vi "Autonomous Independent.vi"   [LabVIEW 2017] (continued)
                  n1739 = call "PID Distance.vi"("Distance"=225.0, "Angle"=0.0, "RightEncoder"=w5983, "LeftEncoder"=w5984, "GyroDevRef"=w5985, "RobotDriveDevRef"=w5986) -> ("RightEncoder 2"=w5987:T11, "LeftEncoder 2"=w5988:T11, "GyroDevRef 2"=w5989:T8, "RobotDriveDevRef 2"=w5990:T1)  [unwired: 2 in]
                }
                frame #1 {
                  n1740 = call "PID turning.vi"("Angle"=-90.0, "GyroDevRef"=w6002, "RobotDriveDevRef"=w6001) -> ("GyroDevRef 2"=w5999:T8, "RobotDriveDevRef 2"=w6000:T1)  [unwired: 7 in]
                }
                frame #2 {
                  n1741 = call <vilib>:"WPI_EncoderReset.vi"("EncoderDevRef"=w6011) -> ("EncoderDevRef"=w6009:T11)  [unwired: 9 in, 1 out]
                  n1742 = Wait (ms)(milliseconds to wait=u32 10) -> ()  [unwired: 1 out]
                  n1743 = call <vilib>:"WPI_EncoderReset.vi"("EncoderDevRef"=w6012) -> ("EncoderDevRef"=w6010:T11)  [unwired: 9 in, 1 out]
                }
                frame #3 {
                  n1744 = global read "Robot Global Data.vi" "Axes"() -> (w6024:dbl[])
                  n1745 = call "PID Distance.vi"("Distance"=199.0, "Angle"=-90.0, "RightEncoder"=w6017, "LeftEncoder"=w6018, "GyroDevRef"=w6019, "RobotDriveDevRef"=w6020) -> ("RightEncoder 2"=w6014:T11, "LeftEncoder 2"=w6013:T11, "GyroDevRef 2"=w6016:T8, "RobotDriveDevRef 2"=w6015:T1)  [unwired: 2 in]
                  n1746 = global write "Robot Global Data.vi" "Lift_Position"(2.0) -> ()
                  n1747 = Array To Cluster(array=w6024) -> (cluster=w6023:T15)
                  n1748 = Bundle By Name(cluster=w6023, "Axes[1]"=-1.0) -> (w6022:T15)
                  n1749 = Cluster To Array(cluster=w6022) -> (array=w6021:dbl[])
                  n1750 = global write "Robot Global Data.vi" "Axes"(w6021) -> ()
                }
                frame #4 {
                  n1751 = call "PID turning.vi"("Angle"=0.0, "GyroDevRef"=w6031, "RobotDriveDevRef"=w6032) -> ("GyroDevRef 2"=w6029:T8, "RobotDriveDevRef 2"=w6030:T1)  [unwired: 7 in]
                }
                frame #5 {
                  n1752 = call <vilib>:"WPI_EncoderReset.vi"("EncoderDevRef"=w6037) -> ("EncoderDevRef"=w6040:T11)  [unwired: 9 in, 1 out]
                  n1753 = call <vilib>:"WPI_EncoderReset.vi"("EncoderDevRef"=w6036) -> ("EncoderDevRef"=w6039:T11)  [unwired: 9 in, 1 out]
                }
                frame #6 {
                  n1754 = call "PID Distance.vi"("Distance"=40.0, "Angle"=0.0, "RightEncoder"=w6047, "LeftEncoder"=w6048, "GyroDevRef"=w6050, "RobotDriveDevRef"=w6049) -> ("RightEncoder 2"=w6043:T11, "LeftEncoder 2"=w6044:T11, "GyroDevRef 2"=w6045:T8, "RobotDriveDevRef 2"=w6046:T1)  [unwired: 2 in]
                  n1755 = global write "Robot Global Data.vi" "Lift_Position"(3.0) -> ()
                }
                frame #7 {
                  n1756 = call "PID turning.vi"("Angle"=20.0, "GyroDevRef"=w6054, "RobotDriveDevRef"=w6057) -> ("GyroDevRef 2"=w6053:T8, "RobotDriveDevRef 2"=w6056:T1)  [unwired: 7 in]
                }
                frame #8 {
                  n1757 = call <vilib>:"WPI_EncoderReset.vi"("EncoderDevRef"=w6063) -> ("EncoderDevRef"=w6061:T11)  [unwired: 9 in, 1 out]
                  n1758 = call <vilib>:"WPI_EncoderReset.vi"("EncoderDevRef"=w6062) -> ("EncoderDevRef"=w6060:T11)  [unwired: 9 in, 1 out]
                }
                frame #9 {
                  w6077 = 0.0 ("Left axis value")
                  n1759 = global read "Robot Global Data.vi" "Axes"() -> (w6072:dbl[])
                  n1760 = Wait (ms)(milliseconds to wait=u32 300) -> ()  [unwired: 1 out]
                  n1761 = Array To Cluster(array=w6072) -> (cluster=w6071:T15)
                  n1762 = Bundle By Name(cluster=w6071, "Axes[1]"=0.25) -> (w6074:T15)
                  n1763 = Cluster To Array(cluster=w6074) -> (array=w6073:dbl[])
                  n1764 = call <vilib>:"WPI_RobotDriveTankDrive.vi"("Right axis value"=w6077, "Left axis value"=w6077, "RobotDriveDevRef"=w6076) -> ("RobotDriveDevRef"=w6070:T1)  [unwired: 6 in, 2 out]
                  n1765 = global write "Robot Global Data.vi" "Axes"(w6073) -> ()
                }
                frame #10 {
                  n1766 = global write "Robot Global Data.vi" "Current State"(FALSE ("Current State")) -> ()
                  n1767 = Wait (ms)(milliseconds to wait=u32 400) -> ()  [unwired: 1 out]
                }
                frame #11 {
                  n1768 = global read "Robot Global Data.vi" "Axes"() -> (w6094:dbl[])
                  n1769 = call "PID Distance.vi"("Distance"=-20.0, "Angle"=20.0, "RightEncoder"=w6095, "LeftEncoder"=w6096, "GyroDevRef"=w6084, "RobotDriveDevRef"=w6085) -> ("RightEncoder 2"=w6086:T11, "LeftEncoder 2"=w6087:T11, "GyroDevRef 2"=w6088:T8, "RobotDriveDevRef 2"=w6089:T1)  [unwired: 2 in]
                  n1770 = Array To Cluster(array=w6094) -> (cluster=w6093:T15)
                  n1771 = Bundle By Name(cluster=w6093, "Axes[1]"=-1.0) -> (w6092:T15)
                  n1772 = Cluster To Array(cluster=w6092) -> (array=w6091:dbl[])
                  n1773 = global write "Robot Global Data.vi" "Axes"(w6091) -> ()
                }
                frame #12 {
                  n1774 = global write "Robot Global Data.vi" "Lift_Position"(1.0) -> ()
                }
                frame #13 {
                  n1775 = case shown="\"L\"" w6104 {
                    tunnel: w6108 -> [w6120 w6196 _]
                    tunnel: w6107 -> [w6119 w6195 _]
                    tunnel: w6106 -> [w6118 w6193 _]
                    tunnel: w6105 -> [w6117 w6194 _]
                    frame "R" {
                      n1776 = flat-sequence {
                        tunnel: w6120 -> [w6129]
                        tunnel: w6119 -> [w6128]
                        tunnel: [w6131] -> w6126
                        tunnel: [w6130] -> w6125
                        tunnel: w6126 -> [w6138]
                        tunnel: w6125 -> [w6137]
                        tunnel: [w6138] -> w6121
                        tunnel: [w6137] -> w6122
                        tunnel: [w6135] -> w6123
                        tunnel: [w6134] -> w6124
                        tunnel: w6118 -> [w6133]
                        tunnel: w6117 -> [w6132]
                        tunnel: w6124 -> [w6139]
                        tunnel: w6123 -> [w6140]
                        tunnel: w6122 -> [w6143]
                        tunnel: w6121 -> [w6144]
                        tunnel: [w6142] -> w6116
                        tunnel: [w6141] -> w6114
                        tunnel: [w6140] -> w6112
                        tunnel: [w6139] -> w6110
                        tunnel: w6116 -> [w6172]
                        tunnel: [w6172] -> w6115
                        tunnel: w6114 -> [w6171]
                        tunnel: [w6171] -> w6113
                        tunnel: w6112 -> [w6170]
                        tunnel: [w6168] -> w6111
                        tunnel: w6110 -> [w6169]
                        tunnel: [w6167] -> w6109
                        tunnel: w6115 -> [w6176]
                        tunnel: w6113 -> [w6175]
                        tunnel: w6111 -> [w6174]
                        tunnel: w6109 -> [w6173]
                        frame #0 {
                          n1777 = call "PID turning.vi"("Angle"=170.0, "GyroDevRef"=w6128, "RobotDriveDevRef"=w6129) -> ("GyroDevRef 2"=w6130:T8, "RobotDriveDevRef 2"=w6131:T1)  [unwired: 7 in]
                        }
                        frame #1 {
                          n1778 = call <vilib>:"WPI_EncoderReset.vi"("EncoderDevRef"=w6133) -> ("EncoderDevRef"=w6134:T11)  [unwired: 9 in, 1 out]
                          n1779 = Wait (ms)(milliseconds to wait=u32 10) -> ()  [unwired: 1 out]
                          n1780 = call <vilib>:"WPI_EncoderReset.vi"("EncoderDevRef"=w6132) -> ("EncoderDevRef"=w6135:T11)  [unwired: 9 in, 1 out]
                        }
                        frame #2 {
                          n1781 = global read "Robot Global Data.vi" "Axes"() -> (w6151:dbl[])
                          n1782 = Wait (ms)(milliseconds to wait=u32 400) -> ()  [unwired: 1 out]
                          n1783 = Array To Cluster(array=w6151) -> (cluster=w6152:T15)
                          n1784 = global read "Robot Global Data.vi" "PIXY Output"() -> (w6145:T16)
                          n1785 = Bundle By Name(cluster=w6152, "Axes[1]"=1.0) -> (w6153:T15)
                          n1786 = Unbundle By Name(w6145) -> ("SIGNATURE NUMBER"=w6148:u16)
                          n1787 = global read "Robot Global Data.vi" "Cube Signature"() -> (w6147:dbl)
                          n1788 = Equal?(x=w6148, y=w6147) -> (x = y?=w6146:bool)
                          n1789 = Cluster To Array(cluster=w6153) -> (array=w6154:dbl[])
                          n1790 = global write "Robot Global Data.vi" "Axes"(w6154) -> ()
                          n1791 = case shown="False" w6146 {
                            tunnel: [w6161 w6164] -> w6141
                            tunnel: [w6162 w6163] -> w6142
                            tunnel: w6144 -> [w6156 w6163]
                            tunnel: w6143 -> [w6155 w6164]
                            frame True {
                              n1792 = call <vilib>:"WPI_GyroGetAngle.vi"("GyroDevRef"=w6155) -> ("Angle"=w6160:dbl, "GyroDevRef"=w6161:T8)  [unwired: 6 in, 3 out]
                              n1793 = In Range and Coerce(upper limit=170.0, x=w6160, lower limit=110.0) -> (coerced(x)=w6159:dbl)  [unwired: 1 out]
                              n1794 = global write "Robot Global Data.vi" "Tracked Angle"(w6159) -> ()
                              n1795 = call "PID vision.vi"("RobotDriveDevRef in"=w6156) -> ("RobotDriveDevRef out"=w6162:T1)  [unwired: 9 in, 1 out]
                            }
                            frame False {
                              n1796 = global write "Robot Global Data.vi" "Tracked Angle"(170.0) -> ()
                            }
                          }
                        }
                        frame #3 {
                          n1797 = call <vilib>:"WPI_EncoderReset.vi"("EncoderDevRef"=w6169) -> ("EncoderDevRef"=w6167:T11)  [unwired: 9 in, 1 out]
                          n1798 = Wait (ms)(milliseconds to wait=u32 10) -> ()  [unwired: 1 out]
                          n1799 = call <vilib>:"WPI_EncoderReset.vi"("EncoderDevRef"=w6170) -> ("EncoderDevRef"=w6168:T11)  [unwired: 9 in, 1 out]
                        }
                        frame #4 {
                          n1800 = global read "Robot Global Data.vi" "Tracked Angle"() -> (w6177:dbl)
                          n1801 = call "PID Distance.vi"("Distance"=50.0, "Angle"=w6177, "RightEncoder"=w6173, "LeftEncoder"=w6174, "GyroDevRef"=w6175, "RobotDriveDevRef"=w6176) -> ()  [unwired: 2 in, 4 out]
                        }
                        frame #5 {
                          n1802 = global write "Robot Global Data.vi" "Current State"(TRUE ("Current State")) -> ()
                          n1803 = Wait (ms)(milliseconds to wait=u32 300) -> ()  [unwired: 1 out]
                        }
                      }
                    }
                    frame "L" {
                      n1804 = flat-sequence {
                        tunnel: w6196 -> [w6213]
                        tunnel: w6195 -> [w6212]
                        tunnel: [w6215] -> w6210
                        tunnel: [w6214] -> w6209
                        tunnel: w6210 -> [w6222]
                        tunnel: w6209 -> [w6221]
                        tunnel: [w6222] -> w6205
                        tunnel: [w6221] -> w6206
                        tunnel: [w6219] -> w6207
                        tunnel: [w6218] -> w6208
                        tunnel: w6193 -> [w6217]
                        tunnel: w6194 -> [w6216]
                        tunnel: w6208 -> [w6223]
                        tunnel: w6207 -> [w6224]
                        tunnel: w6206 -> [w6227]
                        tunnel: w6205 -> [w6228]
                        tunnel: [w6226] -> w6204
                        tunnel: [w6225] -> w6203
                        tunnel: [w6224] -> w6202
                        tunnel: [w6223] -> w6201
                        tunnel: w6204 -> [w6256]
                        tunnel: [w6256] -> w6200
                        tunnel: w6203 -> [w6255]
                        tunnel: [w6255] -> w6199
                        tunnel: w6202 -> [w6254]
                        tunnel: [w6252] -> w6198
                        tunnel: w6201 -> [w6253]
                        tunnel: [w6251] -> w6197
                        tunnel: w6200 -> [w6264]
                        tunnel: w6199 -> [w6263]
                        tunnel: w6198 -> [w6262]
                        tunnel: w6197 -> [w6261]
                        tunnel: [w6260] -> w6190
                        tunnel: [w6259] -> w6187
                        tunnel: [w6258] -> w6184
                        tunnel: [w6257] -> w6181
                        tunnel: [w6270] -> w6191
                        tunnel: w6190 -> [w6270]
                        tunnel: [w6269] -> w6188
                        tunnel: w6187 -> [w6269]
                        tunnel: [w6268] -> w6185
                        tunnel: w6184 -> [w6268]
                        tunnel: [w6267] -> w6182
                        tunnel: w6181 -> [w6267]
                        tunnel: [w6276] -> w6192
                        tunnel: w6191 -> [w6276]
                        tunnel: [w6275] -> w6189
                        tunnel: w6188 -> [w6275]
                        tunnel: [w6274] -> w6186
                        tunnel: w6185 -> [w6274]
                        tunnel: [w6273] -> w6183
                        tunnel: w6182 -> [w6273]
                        tunnel: w6192 -> [w6287]
                        tunnel: w6189 -> [w6286]
                        tunnel: w6186 -> [w6285]
                        tunnel: w6183 -> [w6284]
                        frame #0 {
                          n1805 = call "PID turning.vi"("Angle"=170.0, "GyroDevRef"=w6212, "RobotDriveDevRef"=w6213) -> ("GyroDevRef 2"=w6214:T8, "RobotDriveDevRef 2"=w6215:T1)  [unwired: 7 in]
                        }
                        frame #1 {
                          n1806 = call <vilib>:"WPI_EncoderReset.vi"("EncoderDevRef"=w6217) -> ("EncoderDevRef"=w6218:T11)  [unwired: 9 in, 1 out]
                          n1807 = Wait (ms)(milliseconds to wait=u32 10) -> ()  [unwired: 1 out]
                          n1808 = call <vilib>:"WPI_EncoderReset.vi"("EncoderDevRef"=w6216) -> ("EncoderDevRef"=w6219:T11)  [unwired: 9 in, 1 out]
                        }
                        frame #2 {
                          n1809 = global read "Robot Global Data.vi" "Axes"() -> (w6235:dbl[])
                          n1810 = Wait (ms)(milliseconds to wait=u32 400) -> ()  [unwired: 1 out]
                          n1811 = Array To Cluster(array=w6235) -> (cluster=w6236:T15)
                          n1812 = global read "Robot Global Data.vi" "PIXY Output"() -> (w6229:T16)
                          n1813 = Bundle By Name(cluster=w6236, "Axes[1]"=1.0) -> (w6237:T15)
                          n1814 = Unbundle By Name(w6229) -> ("SIGNATURE NUMBER"=w6232:u16)
                          n1815 = global read "Robot Global Data.vi" "Cube Signature"() -> (w6231:dbl)
                          n1816 = Equal?(x=w6232, y=w6231) -> (x = y?=w6230:bool)
                          n1817 = Cluster To Array(cluster=w6237) -> (array=w6238:dbl[])
                          n1818 = global write "Robot Global Data.vi" "Axes"(w6238) -> ()
                          n1819 = case shown="True" w6230 {
                            tunnel: [w6245 w6248] -> w6225
                            tunnel: [w6246 w6247] -> w6226
                            tunnel: w6228 -> [w6240 w6247]
                            tunnel: w6227 -> [w6239 w6248]
                            frame True {
                              n1820 = call <vilib>:"WPI_GyroGetAngle.vi"("GyroDevRef"=w6239) -> ("Angle"=w6244:dbl, "GyroDevRef"=w6245:T8)  [unwired: 6 in, 3 out]
                              n1821 = In Range and Coerce(upper limit=170.0, x=w6244, lower limit=155.0) -> (coerced(x)=w6243:dbl)  [unwired: 1 out]
                              n1822 = global write "Robot Global Data.vi" "Tracked Angle"(w6243) -> ()
                              n1823 = call "PID vision.vi"("RobotDriveDevRef in"=w6240) -> ("RobotDriveDevRef out"=w6246:T1)  [unwired: 9 in, 1 out]
                            }
                            frame False {
                              n1824 = global write "Robot Global Data.vi" "Tracked Angle"(170.0) -> ()
                            }
                          }
                        }
                        frame #3 {
                          n1825 = call <vilib>:"WPI_EncoderReset.vi"("EncoderDevRef"=w6253) -> ("EncoderDevRef"=w6251:T11)  [unwired: 9 in, 1 out]
                          n1826 = Wait (ms)(milliseconds to wait=u32 10) -> ()  [unwired: 1 out]
                          n1827 = call <vilib>:"WPI_EncoderReset.vi"("EncoderDevRef"=w6254) -> ("EncoderDevRef"=w6252:T11)  [unwired: 9 in, 1 out]
                        }
                        frame #4 {
                          n1828 = global read "Robot Global Data.vi" "Tracked Angle"() -> (w6265:dbl)
                          n1829 = call "PID Distance.vi"("Distance"=50.0, "Angle"=w6265, "RightEncoder"=w6261, "LeftEncoder"=w6262, "GyroDevRef"=w6263, "RobotDriveDevRef"=w6264) -> ("RightEncoder 2"=w6257:T11, "LeftEncoder 2"=w6258:T11, "GyroDevRef 2"=w6259:T8, "RobotDriveDevRef 2"=w6260:T1)  [unwired: 2 in]
                        }
                        frame #5 {
                          n1830 = global write "Robot Global Data.vi" "Current State"(TRUE ("Current State")) -> ()
                          n1831 = Wait (ms)(milliseconds to wait=u32 500) -> ()  [unwired: 1 out]
                        }
                        frame #6 {
                          n1832 = global read "Robot Global Data.vi" "Axes"() -> (w6282:dbl[])
                          n1833 = global write "Robot Global Data.vi" "Lift_Position"(2.0) -> ()
                          n1834 = Wait (ms)(milliseconds to wait=u32 400) -> ()  [unwired: 1 out]
                          n1835 = Array To Cluster(array=w6282) -> (cluster=w6281:T15)
                          n1836 = Bundle By Name(cluster=w6281, "Axes[1]"=-1.0) -> (w6280:T15)
                          n1837 = Cluster To Array(cluster=w6280) -> (array=w6279:dbl[])
                          n1838 = global write "Robot Global Data.vi" "Axes"(w6279) -> ()
                        }
                        frame #7 {
                          n1839 = global read "Robot Global Data.vi" "Tracked Angle"() -> (w6288:dbl)
                          n1840 = call "PID Distance.vi"("Distance"=66.0, "Angle"=w6288, "RightEncoder"=w6284, "LeftEncoder"=w6285, "GyroDevRef"=w6286, "RobotDriveDevRef"=w6287) -> ()  [unwired: 2 in, 4 out]
                        }
                        frame #8 {
                          n1841 = global read "Robot Global Data.vi" "Axes"() -> (w6295:dbl[])
                          n1842 = Wait (ms)(milliseconds to wait=u32 200) -> ()  [unwired: 1 out]
                          n1843 = Array To Cluster(array=w6295) -> (cluster=w6294:T15)
                          n1844 = Bundle By Name(cluster=w6294, "Axes[1]"=0.5) -> (w6293:T15)
                          n1845 = Cluster To Array(cluster=w6293) -> (array=w6292:dbl[])
                          n1846 = global write "Robot Global Data.vi" "Axes"(w6292) -> ()
                        }
                        frame #9 {
                          n1847 = global write "Robot Global Data.vi" "Current State"(FALSE ("Current State")) -> ()
                        }
                      }
                    }
                    frame Default {
                    }
                  }
                }
              }
            }
            frame "R" {
              n1848 = flat-sequence {
                tunnel: [w6362] -> w6350
                tunnel: [w6361] -> w6351
                tunnel: [w6359] -> w6352
                tunnel: [w6360] -> w6353
                tunnel: w6309 -> [w6358]
                tunnel: w6308 -> [w6357]
                tunnel: w6307 -> [w6356]
                tunnel: w6306 -> [w6355]
                tunnel: [w6382] -> w6349
                tunnel: w6353 -> [w6378]
                tunnel: w6352 -> [w6379]
                tunnel: w6351 -> [w6381]
                tunnel: w6350 -> [w6383]
                tunnel: [w6380] -> w6348
                tunnel: [w6379] -> w6347
                tunnel: [w6378] -> w6346
                tunnel: w6349 -> [w6393]
                tunnel: [w6393] -> w6345
                tunnel: w6348 -> [w6392]
                tunnel: [w6392] -> w6344
                tunnel: [w6391] -> w6343
                tunnel: [w6390] -> w6342
                tunnel: w6347 -> [w6388]
                tunnel: w6346 -> [w6387]
                tunnel: w6345 -> [w6399]
                tunnel: [w6397] -> w6341
                tunnel: w6344 -> [w6398]
                tunnel: [w6396] -> w6340
                tunnel: w6343 -> [w6401]
                tunnel: w6342 -> [w6400]
                tunnel: [w6395] -> w6339
                tunnel: [w6394] -> w6338
                tunnel: w6341 -> [w6408]
                tunnel: [w6407] -> w6337
                tunnel: [w6406] -> w6336
                tunnel: w6340 -> [w6406]
                tunnel: [w6405] -> w6335
                tunnel: w6339 -> [w6405]
                tunnel: [w6404] -> w6334
                tunnel: w6338 -> [w6404]
                tunnel: [w6419] -> w6333
                tunnel: w6337 -> [w6419]
                tunnel: [w6418] -> w6332
                tunnel: w6336 -> [w6418]
                tunnel: [w6417] -> w6331
                tunnel: w6335 -> [w6417]
                tunnel: [w6416] -> w6330
                tunnel: w6334 -> [w6416]
                tunnel: w6333 -> [w6424]
                tunnel: w6332 -> [w6425]
                tunnel: [w6425] -> w6329
                tunnel: [w6424] -> w6328
                tunnel: [w6423] -> w6327
                tunnel: w6331 -> [w6423]
                tunnel: [w6422] -> w6326
                tunnel: w6330 -> [w6422]
                tunnel: [w6438] -> w6325
                tunnel: w6329 -> [w6440]
                tunnel: w6328 -> [w6439]
                tunnel: w6327 -> [w6435]
                tunnel: w6326 -> [w6434]
                tunnel: [w6433] -> w6324
                tunnel: [w6432] -> w6323
                tunnel: [w6431] -> w6322
                tunnel: w6325 -> [w6447]
                tunnel: w6324 -> [w6446]
                tunnel: [w6445] -> w6304
                tunnel: w6323 -> [w6445]
                tunnel: [w6444] -> w6302
                tunnel: w6322 -> [w6444]
                tunnel: [w6443] -> w6300
                tunnel: [w6442] -> w6298
                tunnel: w6304 -> [w6454]
                tunnel: [w6450] -> w6303
                tunnel: w6302 -> [w6453]
                tunnel: [w6449] -> w6301
                tunnel: w6300 -> [w6456]
                tunnel: [w6452] -> w6299
                tunnel: w6298 -> [w6455]
                tunnel: [w6451] -> w6297
                tunnel: w6303 -> [w6482]
                tunnel: w6301 -> [w6481]
                tunnel: [w6479] -> w6321
                tunnel: w6299 -> [w6479]
                tunnel: [w6478] -> w6320
                tunnel: w6297 -> [w6478]
                tunnel: [w6477] -> w6319
                tunnel: [w6476] -> w6318
                tunnel: w6321 -> [w6497]
                tunnel: w6320 -> [w6496]
                tunnel: w6319 -> [w6495]
                tunnel: w6318 -> [w6494]
                tunnel: [w6493] -> w6317
                tunnel: [w6492] -> w6316
                tunnel: [w6491] -> w6315
                tunnel: [w6490] -> w6314
                tunnel: [w6502] -> w6313
                tunnel: [w6499] -> w6312
                tunnel: [w6501] -> w6311
                tunnel: [w6500] -> w6310
                tunnel: w6314 -> [w6499]
                tunnel: w6315 -> [w6500]
                tunnel: w6316 -> [w6501]
                tunnel: w6317 -> [w6502]
                tunnel: w6313 -> [w6509]
                tunnel: w6312 -> [w6508]
                tunnel: w6311 -> [w6507]
                tunnel: w6310 -> [w6506]
                tunnel: w6305 -> [w6505]
                frame #0 {
                  n1849 = while {
                    tunnel: [w6367] -> w6354
                    stop <- w6366 stop-if-true
                    w6370 = 100.0 ("y")
                    w6373 = 20.0 ("y")
                    n1850 = global read "Robot Global Data.vi" "Distance 2"() -> (w6368:dbl)
                    n1851 = global read "Robot Global Data.vi" "Distance"() -> (w6369:dbl)
                    n1852 = Greater?(x=w6369, y=w6373) -> (0:w6375:bool)
                    n1853 = Greater?(x=w6368, y=w6373) -> (0:w6374:bool)
                    n1854 = Greater?(x=w6369, y=w6370) -> (0:w6372:bool)
                    n1855 = Greater?(x=w6368, y=w6370) -> (0:w6371:bool)
                    n1856 = Or(x=w6375, y=w6374) -> (x .or. y?=w6365:bool)
                    n1857 = Or(x=w6372, y=w6371) -> (x .or. y?=w6366:bool)
                    n1858 = global write "Robot Global Data.vi" "Raise_Mast"(w6365) -> ()
                    n1859 = case shown="True" w6366 {
                      tunnel: [0.0 2.0] -> w6367
                      frame False {
                      }
                      frame True {
                      }
                    }
                  }
                  n1860 = call "PID Distance.vi"("Distance"=295.0, "Angle"=2.0, "RightEncoder"=w6355, "LeftEncoder"=w6356, "GyroDevRef"=w6357, "RobotDriveDevRef"=w6358) -> ("RightEncoder 2"=w6359:T11, "LeftEncoder 2"=w6360:T11, "GyroDevRef 2"=w6361:T8, "RobotDriveDevRef 2"=w6362:T1)  [unwired: 2 in]
                  n1861 = global write "Robot Global Data.vi" "Lift_Position"(w6354) -> ()
                }
                frame #1 {
                  n1862 = call "PID turning.vi"("Angle"=-90.0, "GyroDevRef"=w6381, "RobotDriveDevRef"=w6383) -> ("GyroDevRef 2"=w6380:T8, "RobotDriveDevRef 2"=w6382:T1)  [unwired: 7 in]
                  n1863 = global write "Robot Global Data.vi" "Lift_Position"(3.0) -> ()
                  n1864 = global write "Robot Global Data.vi" "Raise_Mast"(TRUE ("Current State")) -> ()
                }
                frame #2 {
                  n1865 = call <vilib>:"WPI_EncoderReset.vi"("EncoderDevRef"=w6387) -> ("EncoderDevRef"=w6390:T11)  [unwired: 9 in, 1 out]
                  n1866 = Wait (ms)(milliseconds to wait=u32 100) -> ()  [unwired: 1 out]
                  n1867 = call <vilib>:"WPI_EncoderReset.vi"("EncoderDevRef"=w6388) -> ("EncoderDevRef"=w6391:T11)  [unwired: 9 in, 1 out]
                }
                frame #3 {
                  n1868 = call "PID Distance.vi"("Distance"=25.0, "Angle"=-90.0, "RightEncoder"=w6401, "LeftEncoder"=w6400, "GyroDevRef"=w6398, "RobotDriveDevRef"=w6399) -> ("RightEncoder 2"=w6394:T11, "LeftEncoder 2"=w6395:T11, "GyroDevRef 2"=w6396:T8, "RobotDriveDevRef 2"=w6397:T1)  [unwired: 2 in]
                }
                frame #4 {
                  w6409 = 0.0 ("Left axis value")
                  n1869 = global read "Robot Global Data.vi" "Axes"() -> (w6412:dbl[])
                  n1870 = Wait (ms)(milliseconds to wait=u32 500) -> ()  [unwired: 1 out]
                  n1871 = Array To Cluster(array=w6412) -> (cluster=w6411:T15)
                  n1872 = Bundle By Name(cluster=w6411, "Axes[1]"=0.25) -> (w6414:T15)
                  n1873 = Cluster To Array(cluster=w6414) -> (array=w6413:dbl[])
                  n1874 = call <vilib>:"WPI_RobotDriveTankDrive.vi"("Right axis value"=w6409, "Left axis value"=w6409, "RobotDriveDevRef"=w6408) -> ("RobotDriveDevRef"=w6407:T1)  [unwired: 6 in, 2 out]
                  n1875 = global write "Robot Global Data.vi" "Axes"(w6413) -> ()
                }
                frame #5 {
                  n1876 = global write "Robot Global Data.vi" "Current State"(FALSE ("Current State")) -> ()
                  n1877 = Wait (ms)(milliseconds to wait=u32 400) -> ()  [unwired: 1 out]
                }
                frame #6 {
                  n1878 = global read "Robot Global Data.vi" "Axes"() -> (w6427:dbl[])
                  n1879 = Array To Cluster(array=w6427) -> (cluster=w6426:T15)
                  n1880 = Bundle By Name(cluster=w6426, "Axes[1]"=-1.0) -> (w6429:T15)
                  n1881 = Cluster To Array(cluster=w6429) -> (array=w6428:dbl[])
                  n1882 = global write "Robot Global Data.vi" "Axes"(w6428) -> ()
                }
                frame #7 {
                  n1883 = call "PID Distance.vi"("Distance"=18.0, "Angle"=-90.0, "RightEncoder"=w6434, "LeftEncoder"=w6435, "GyroDevRef"=w6440, "RobotDriveDevRef"=w6439) -> ("RightEncoder 2"=w6431:T11, "LeftEncoder 2"=w6432:T11, "GyroDevRef 2"=w6433:T8, "RobotDriveDevRef 2"=w6438:T1)  [unwired: 2 in]
                }
                frame #8 {
                  n1884 = global write "Robot Global Data.vi" "Lift_Position"(1.0) -> ()
                  n1885 = call "PID turning.vi"("Angle"=-155.0, "GyroDevRef"=w6446, "RobotDriveDevRef"=w6447) -> ("GyroDevRef 2"=w6442:T8, "RobotDriveDevRef 2"=w6443:T1)  [unwired: 7 in]
                }
                frame #9 {
                  n1886 = global read "Robot Global Data.vi" "PIXY Output"() -> (w6460:T16)
                  n1887 = Unbundle By Name(w6460) -> ("SIGNATURE NUMBER"=w6459:u16)
                  n1888 = global read "Robot Global Data.vi" "Cube Signature"() -> (w6458:dbl)
                  n1889 = Equal?(x=w6459, y=w6458) -> (x = y?=w6457:bool)
                  n1890 = case shown="True" w6457 {
                    tunnel: [w6467 w6471] -> w6449
                    tunnel: [w6466 w6472] -> w6450
                    tunnel: [w6465 w6473] -> w6451
                    tunnel: [w6469 w6474] -> w6452
                    tunnel: w6454 -> [w6466 w6472]
                    tunnel: w6453 -> [w6467 w6471]
                    tunnel: w6455 -> [w6468 w6473]
                    tunnel: w6456 -> [w6470 w6474]
                    frame True {
                      n1891 = call <vilib>:"WPI_GyroGetAngle.vi"("GyroDevRef"=w6468) -> ("Angle"=w6464:dbl, "GyroDevRef"=w6465:T8)  [unwired: 6 in, 3 out]
                      n1892 = In Range and Coerce(upper limit=-150.0, x=w6464, lower limit=-170.0) -> (coerced(x)=w6463:dbl)  [unwired: 1 out]
                      n1893 = global write "Robot Global Data.vi" "Tracked Angle"(w6463) -> ()
                      n1894 = call "PID vision.vi"("RobotDriveDevRef in"=w6470) -> ("RobotDriveDevRef out"=w6469:T1)  [unwired: 9 in, 1 out]
                    }
                    frame False {
                      n1895 = global write "Robot Global Data.vi" "Tracked Angle"(-150.0) -> ()
                    }
                  }
                }
                frame #10 {
                  n1896 = call <vilib>:"WPI_EncoderReset.vi"("EncoderDevRef"=w6482) -> ("EncoderDevRef"=w6477:T11)  [unwired: 9 in, 1 out]
                  n1897 = Wait (ms)(milliseconds to wait=u32 10) -> ()  [unwired: 1 out]
                  n1898 = call <vilib>:"WPI_EncoderReset.vi"("EncoderDevRef"=w6481) -> ("EncoderDevRef"=w6476:T11)  [unwired: 9 in, 1 out]
                }
                frame #11 {
                  n1899 = global write "Robot Global Data.vi" "Lift_Position"(0.0) -> ()
                  n1900 = global read "Robot Global Data.vi" "Axes"() -> (w6487:dbl[])
                  n1901 = Array To Cluster(array=w6487) -> (cluster=w6486:T15)
                  n1902 = global read "Robot Global Data.vi" "Tracked Angle"() -> (w6484:dbl)
                  n1903 = Bundle By Name(cluster=w6486, "Axes[1]"=1.0) -> (w6489:T15)
                  n1904 = call "PID Distance.vi"("Distance"=106.0, "Angle"=w6484, "RightEncoder"=w6494, "LeftEncoder"=w6495, "GyroDevRef"=w6496, "RobotDriveDevRef"=w6497) -> ("RightEncoder 2"=w6490:T11, "LeftEncoder 2"=w6491:T11, "GyroDevRef 2"=w6492:T8, "RobotDriveDevRef 2"=w6493:T1)  [unwired: 2 in]
                  n1905 = Cluster To Array(cluster=w6489) -> (array=w6488:dbl[])
                  n1906 = global write "Robot Global Data.vi" "Axes"(w6488) -> ()
                }
                frame #12 {
                  n1907 = global write "Robot Global Data.vi" "Current State"(TRUE ("Current State")) -> ()
                  n1908 = Wait (ms)(milliseconds to wait=u32 750) -> ()  [unwired: 1 out]
                }
                frame #13 {
                  n1909 = case shown="\"L\"" w6505 {
                    tunnel: w6509 -> [w6513 w6566 _]
                    tunnel: w6508 -> [w6510 w6565 _]
                    tunnel: w6507 -> [w6512 w6564 _]
                    tunnel: w6506 -> [w6511 w6563 _]
                    frame "R" {
                      n1910 = flat-sequence {
                        tunnel: w6513 -> [w6525]
                        tunnel: w6512 -> [w6524]
                        tunnel: w6510 -> [w6522]
                        tunnel: w6511 -> [w6523]
                        frame #0 {
                          n1911 = global read "Robot Global Data.vi" "Axes"() -> (w6518:dbl[])
                          n1912 = global write "Robot Global Data.vi" "Lift_Position"(2.0) -> ()
                          n1913 = Wait (ms)(milliseconds to wait=u32 250) -> ()  [unwired: 1 out]
                          n1914 = Array To Cluster(array=w6518) -> (cluster=w6517:T15)
                          n1915 = Bundle By Name(cluster=w6517, "Axes[1]"=-1.0) -> (w6520:T15)
                          n1916 = Cluster To Array(cluster=w6520) -> (array=w6519:dbl[])
                          n1917 = global write "Robot Global Data.vi" "Axes"(w6519) -> ()
                        }
                        frame #1 {
                          n1918 = global read "Robot Global Data.vi" "Tracked Angle"() -> (w6521:dbl)
                          n1919 = call "PID Distance.vi"("Distance"=119.0, "Angle"=w6521, "RightEncoder"=w6522, "LeftEncoder"=w6523, "GyroDevRef"=w6524, "RobotDriveDevRef"=w6525) -> ()  [unwired: 2 in, 4 out]
                        }
                        frame #2 {
                          n1920 = global read "Robot Global Data.vi" "Axes"() -> (w6530:dbl[])
                          n1921 = Wait (ms)(milliseconds to wait=u32 200) -> ()  [unwired: 1 out]
                          n1922 = Array To Cluster(array=w6530) -> (cluster=w6529:T15)
                          n1923 = Bundle By Name(cluster=w6529, "Axes[1]"=0.5) -> (w6532:T15)
                          n1924 = Cluster To Array(cluster=w6532) -> (array=w6531:dbl[])
                          n1925 = global write "Robot Global Data.vi" "Axes"(w6531) -> ()
                        }
                        frame #3 {
                          n1926 = global write "Robot Global Data.vi" "Current State"(FALSE ("Current State")) -> ()
                          n1927 = Wait (ms)(milliseconds to wait=u32 500) -> ()  [unwired: 1 out]
                        }
                      }
                    }
                    frame "L" {
                      n1928 = flat-sequence {
                        tunnel: w6566 -> [w6577]
                        tunnel: w6565 -> [w6582]
                        tunnel: w6564 -> [w6576]
                        tunnel: w6563 -> [w6575]
                        tunnel: [w6581] -> w6562
                        tunnel: [w6580] -> w6561
                        tunnel: [w6579] -> w6559
                        tunnel: [w6578] -> w6557
                        tunnel: w6562 -> [w6590]
                        tunnel: w6561 -> [w6589]
                        tunnel: [w6588] -> w6560
                        tunnel: w6559 -> [w6588]
                        tunnel: [w6587] -> w6558
                        tunnel: w6557 -> [w6587]
                        tunnel: [w6586] -> w6555
                        tunnel: [w6585] -> w6553
                        tunnel: w6560 -> [w6597]
                        tunnel: w6558 -> [w6596]
                        tunnel: [w6595] -> w6556
                        tunnel: w6555 -> [w6595]
                        tunnel: [w6594] -> w6554
                        tunnel: w6553 -> [w6594]
                        tunnel: [w6593] -> w6552
                        tunnel: [w6592] -> w6551
                        tunnel: w6556 -> [w6607]
                        tunnel: w6554 -> [w6606]
                        tunnel: w6552 -> [w6605]
                        tunnel: w6551 -> [w6604]
                        tunnel: [w6603] -> w6550
                        tunnel: [w6602] -> w6549
                        tunnel: [w6600] -> w6548
                        tunnel: [w6599] -> w6547
                        tunnel: [w6613] -> w6546
                        tunnel: [w6612] -> w6545
                        tunnel: [w6611] -> w6544
                        tunnel: [w6610] -> w6543
                        tunnel: w6547 -> [w6610]
                        tunnel: w6548 -> [w6611]
                        tunnel: w6549 -> [w6612]
                        tunnel: w6550 -> [w6613]
                        tunnel: [w6623] -> w6536
                        tunnel: w6546 -> [w6623]
                        tunnel: [w6622] -> w6538
                        tunnel: w6545 -> [w6622]
                        tunnel: [w6621] -> w6540
                        tunnel: w6544 -> [w6621]
                        tunnel: [w6620] -> w6542
                        tunnel: w6543 -> [w6620]
                        tunnel: w6542 -> [w6635]
                        tunnel: [w6635] -> w6541
                        tunnel: w6540 -> [w6634]
                        tunnel: [w6634] -> w6539
                        tunnel: w6538 -> [w6633]
                        tunnel: [w6633] -> w6537
                        tunnel: w6536 -> [w6632]
                        tunnel: [w6632] -> w6535
                        tunnel: w6541 -> [w6636]
                        tunnel: w6539 -> [w6637]
                        tunnel: w6537 -> [w6638]
                        tunnel: w6535 -> [w6639]
                        frame #0 {
                          n1929 = global read "Robot Global Data.vi" "Axes"() -> (w6571:dbl[])
                          n1930 = global write "Robot Global Data.vi" "Lift_Position"(2.0) -> ()
                          n1931 = Wait (ms)(milliseconds to wait=u32 250) -> ()  [unwired: 1 out]
                          n1932 = Array To Cluster(array=w6571) -> (cluster=w6570:T15)
                          n1933 = Bundle By Name(cluster=w6570, "Axes[1]"=-1.0) -> (w6573:T15)
                          n1934 = Cluster To Array(cluster=w6573) -> (array=w6572:dbl[])
                          n1935 = global write "Robot Global Data.vi" "Axes"(w6572) -> ()
                        }
                        frame #1 {
                          n1936 = global read "Robot Global Data.vi" "Tracked Angle"() -> (w6574:dbl)
                          n1937 = call "PID Distance.vi"("Distance"=-20.0, "Angle"=w6574, "RightEncoder"=w6582, "LeftEncoder"=w6575, "GyroDevRef"=w6576, "RobotDriveDevRef"=w6577) -> ("RightEncoder 2"=w6578:T11, "LeftEncoder 2"=w6579:T11, "GyroDevRef 2"=w6580:T8, "RobotDriveDevRef 2"=w6581:T1)  [unwired: 2 in]
                        }
                        frame #2 {
                          n1938 = call "PID turning.vi"("Angle"=-90.0, "GyroDevRef"=w6589, "RobotDriveDevRef"=w6590) -> ("GyroDevRef 2"=w6585:T8, "RobotDriveDevRef 2"=w6586:T1)  [unwired: 7 in]
                          n1939 = global write "Robot Global Data.vi" "Lift_Position"(3.0) -> ()
                        }
                        frame #3 {
                          n1940 = call <vilib>:"WPI_EncoderReset.vi"("EncoderDevRef"=w6597) -> ("EncoderDevRef"=w6593:T11)  [unwired: 9 in, 1 out]
                          n1941 = Wait (ms)(milliseconds to wait=u32 10) -> ()  [unwired: 1 out]
                          n1942 = call <vilib>:"WPI_EncoderReset.vi"("EncoderDevRef"=w6596) -> ("EncoderDevRef"=w6592:T11)  [unwired: 9 in, 1 out]
                        }
                        frame #4 {
                          n1943 = global write "Robot Global Data.vi" "Lift_Position"(3.0) -> ()
                          n1944 = call "PID Distance.vi"("Distance"=30.0, "Angle"=-90.0, "RightEncoder"=w6604, "LeftEncoder"=w6605, "GyroDevRef"=w6606, "RobotDriveDevRef"=w6607) -> ("RightEncoder 2"=w6599:T11, "LeftEncoder 2"=w6600:T11, "GyroDevRef 2"=w6602:T8, "RobotDriveDevRef 2"=w6603:T1)  [unwired: 2 in]
                        }
                        frame #5 {
                          n1945 = global read "Robot Global Data.vi" "Axes"() -> (w6617:dbl[])
                          n1946 = Wait (ms)(milliseconds to wait=u32 500) -> ()  [unwired: 1 out]
                          n1947 = Array To Cluster(array=w6617) -> (cluster=w6616:T15)
                          n1948 = Bundle By Name(cluster=w6616, "Axes[1]"=0.3) -> (w6619:T15)
                          n1949 = Cluster To Array(cluster=w6619) -> (array=w6618:dbl[])
                          n1950 = global write "Robot Global Data.vi" "Axes"(w6618) -> ()
                        }
                        frame #6 {
                          n1951 = global write "Robot Global Data.vi" "Current State"(FALSE ("Current State")) -> ()
                          n1952 = Wait (ms)(milliseconds to wait=u32 400) -> ()  [unwired: 1 out]
                        }
                        frame #7 {
                          n1953 = global read "Robot Global Data.vi" "Axes"() -> (w6629:dbl[])
                          n1954 = Wait (ms)(milliseconds to wait=u32 250) -> ()  [unwired: 1 out]
                          n1955 = Array To Cluster(array=w6629) -> (cluster=w6628:T15)
                          n1956 = Bundle By Name(cluster=w6628, "Axes[1]"=-1.0) -> (w6631:T15)
                          n1957 = Cluster To Array(cluster=w6631) -> (array=w6630:dbl[])
                          n1958 = global write "Robot Global Data.vi" "Axes"(w6630) -> ()
                        }
                        frame #8 {
                          n1959 = call "PID Distance.vi"("Distance"=0.0, "Angle"=90.0, "RightEncoder"=w6636, "LeftEncoder"=w6637, "GyroDevRef"=w6638, "RobotDriveDevRef"=w6639) -> ()  [unwired: 2 in, 4 out]
                        }
                        frame #9 {
                          n1960 = global write "Robot Global Data.vi" "Lift_Position"(1.0) -> ()
                        }
                      }
                    }
                    frame Default {
                    }
                  }
                }
              }
            }
            frame Default {
              n1961 = flat-sequence {
                tunnel: w6644 -> [w6652]
                tunnel: w6643 -> [w6651]
                tunnel: w6645 -> [w6649]
                tunnel: [w6650] -> w6647
                tunnel: w6646 -> [w6648]
                tunnel: w6647 -> [w6655]
                frame #0 {
                  n1962 = call "PID Distance.vi"("Distance"=90.0, "Angle"=0.0, "RightEncoder"=w6648, "LeftEncoder"=w6649, "GyroDevRef"=w6651, "RobotDriveDevRef"=w6652) -> ("RobotDriveDevRef 2"=w6650:T1)  [unwired: 2 in, 3 out]
                }
                frame #1 {
                  w6656 = 0.0
                  n1963 = call <vilib>:"WPI_RobotDriveTankDrive.vi"("Right axis value"=w6656, "Left axis value"=w6656, "RobotDriveDevRef"=w6655) -> ()  [unwired: 6 in, 3 out]
                }
              }
            }
          }
        }
      }
    }
    frame "Right Scale V2" {
      n1964 = flat-sequence {
        tunnel: w6664 -> [w6693]
        tunnel: w6662 -> [w6691]
        tunnel: w6663 -> [w6690]
        tunnel: [w6689] -> w6668
        tunnel: [w6688] -> w6667
        tunnel: [w6687] -> w6666
        tunnel: [w6686] -> w6665
        tunnel: w6660 -> [w6679]
        tunnel: w6661 -> [w6669]
        tunnel: w6659 -> [w6696]
        tunnel: w6668 -> [w6700]
        tunnel: w6667 -> [w6699]
        tunnel: w6666 -> [w6698]
        tunnel: w6665 -> [w6697]
        tunnel: w6658 -> [w6695]
        tunnel: w6657 -> [w6694]
        frame #0 {
          w6692 = 0.0 ("Left axis value")
          n1965 = global read "Robot Global Data.vi" "Axes"() -> (w6672:dbl[])
          n1966 = Multiply(x=w6679, y=1000.0) -> (x*y=w6680:dbl)
          n1967 = global write "Robot Global Data.vi" "Lift_Position"(0.0) -> ()
          n1968 = global write "Robot Global Data.vi" "Current State"(TRUE ("Current State")) -> ()
          n1969 = global write "Robot Global Data.vi" "Raise_Mast"(FALSE ("Current State")) -> ()
          n1970 = Wait (ms)(milliseconds to wait=u32 100) -> ()  [unwired: 1 out]
          n1971 = Array To Cluster(array=w6672) -> (cluster=w6671:T15)
          n1972 = Bundle By Name(cluster=w6671, "Axes[1]"=-1.0) -> (w6674:T15)
          n1973 = Greater?(x=w6680, y=11000.0) -> (0:w6682:bool)
          n1974 = Equal?(x=w6680, y=0.0) -> (x = y?=w6683:bool)
          n1975 = Or(x=w6682, y=w6683) -> ()  [unwired: 1 out]
          n1976 = Cluster To Array(cluster=w6674) -> (array=w6673:dbl[])
          n1977 = call <vilib>:"WPI_GyroReset.vi"("GyroDevRef"=w6690) -> ("GyroDevRef"=w6686:T8)  [unwired: 9 in, 1 out]
          n1978 = call <vilib>:"WPI_EncoderReset.vi"("EncoderDevRef"=w6669) -> ("EncoderDevRef"=w6688:T11)  [unwired: 9 in, 1 out]
          n1979 = global write "Robot Global Data.vi" "Axes"(w6673) -> ()
          n1980 = call <vilib>:"WPI_EncoderReset.vi"("EncoderDevRef"=w6691) -> ("EncoderDevRef"=w6687:T11)  [unwired: 9 in, 1 out]
          n1981 = call <vilib>:"WPI_RobotDriveTankDrive.vi"("Right axis value"=w6692, "Left axis value"=w6692, "RobotDriveDevRef"=w6693) -> ("RobotDriveDevRef"=w6689:T1)  [unwired: 6 in, 2 out]
        }
        frame #1 {
          n1982 = case shown="\"R\"" w6696 {
            tunnel: w6700 -> [w6711 w7101 w7451]
            tunnel: w6699 -> [w6714 w7098 w7453]
            tunnel: w6698 -> [w6713 w7099 w7452]
            tunnel: w6697 -> [w6712 w7100 w7450]
            tunnel: w6695 -> [w6710 w7097 _]
            tunnel: w6694 -> [w6701 w7089 _]
            frame "L" {
              n1983 = flat-sequence {
                tunnel: [w6766] -> w6758
                tunnel: [w6765] -> w6757
                tunnel: [w6763] -> w6756
                tunnel: [w6764] -> w6755
                tunnel: w6714 -> [w6759]
                tunnel: w6713 -> [w6760]
                tunnel: w6712 -> [w6761]
                tunnel: w6711 -> [w6762]
                tunnel: w6758 -> [w6777]
                tunnel: w6757 -> [w6778]
                tunnel: [w6781] -> w6754
                tunnel: w6756 -> [w6781]
                tunnel: [w6780] -> w6753
                tunnel: w6755 -> [w6780]
                tunnel: [w6775] -> w6752
                tunnel: [w6776] -> w6751
                tunnel: w6754 -> [w6788]
                tunnel: w6753 -> [w6787]
                tunnel: [w6786] -> w6750
                tunnel: [w6785] -> w6749
                tunnel: [w6784] -> w6748
                tunnel: w6752 -> [w6784]
                tunnel: [w6782] -> w6747
                tunnel: w6751 -> [w6782]
                tunnel: w6750 -> [w6793]
                tunnel: w6749 -> [w6794]
                tunnel: w6748 -> [w6795]
                tunnel: [w6791] -> w6746
                tunnel: [w6792] -> w6745
                tunnel: w6747 -> [w6796]
                tunnel: [w6789] -> w6744
                tunnel: [w6790] -> w6743
                tunnel: w6746 -> [w6808]
                tunnel: w6745 -> [w6807]
                tunnel: [w6806] -> w6742
                tunnel: [w6805] -> w6741
                tunnel: [w6811] -> w6740
                tunnel: w6744 -> [w6811]
                tunnel: [w6810] -> w6739
                tunnel: w6743 -> [w6810]
                tunnel: w6742 -> [w6817]
                tunnel: [w6817] -> w6738
                tunnel: [w6816] -> w6737
                tunnel: [w6815] -> w6736
                tunnel: [w6814] -> w6735
                tunnel: w6741 -> [w6814]
                tunnel: w6740 -> [w6813]
                tunnel: w6739 -> [w6812]
                tunnel: w6738 -> [w6825]
                tunnel: [w6822] -> w6734
                tunnel: w6737 -> [w6824]
                tunnel: w6736 -> [w6823]
                tunnel: w6735 -> [w6826]
                tunnel: [w6821] -> w6733
                tunnel: [w6820] -> w6732
                tunnel: [w6819] -> w6731
                tunnel: w6734 -> [w6833]
                tunnel: [w6832] -> w6709
                tunnel: w6733 -> [w6830]
                tunnel: [w6829] -> w6707
                tunnel: w6732 -> [w6835]
                tunnel: [w6835] -> w6705
                tunnel: w6731 -> [w6834]
                tunnel: [w6834] -> w6703
                tunnel: w6709 -> [w6841]
                tunnel: [w6841] -> w6708
                tunnel: w6707 -> [w6840]
                tunnel: [w6840] -> w6706
                tunnel: w6705 -> [w6839]
                tunnel: [w6837] -> w6704
                tunnel: w6703 -> [w6838]
                tunnel: [w6836] -> w6702
                tunnel: w6708 -> [w6852]
                tunnel: [w6846] -> w6730
                tunnel: [w6845] -> w6729
                tunnel: w6706 -> [w6845]
                tunnel: [w6844] -> w6728
                tunnel: w6704 -> [w6844]
                tunnel: [w6843] -> w6727
                tunnel: w6702 -> [w6843]
                tunnel: w6730 -> [w6859]
                tunnel: [w6859] -> w6726
                tunnel: w6729 -> [w6858]
                tunnel: [w6858] -> w6725
                tunnel: w6728 -> [w6857]
                tunnel: [w6857] -> w6724
                tunnel: w6727 -> [w6856]
                tunnel: [w6856] -> w6723
                tunnel: [w6865] -> w6722
                tunnel: [w6864] -> w6721
                tunnel: [w6863] -> w6720
                tunnel: [w6862] -> w6719
                tunnel: w6723 -> [w6871]
                tunnel: w6724 -> [w6872]
                tunnel: w6725 -> [w6860]
                tunnel: w6726 -> [w6861]
                tunnel: w6722 -> [w6879]
                tunnel: [w6879] -> w6718
                tunnel: w6721 -> [w6878]
                tunnel: [w6878] -> w6717
                tunnel: w6720 -> [w6877]
                tunnel: [w6877] -> w6716
                tunnel: w6719 -> [w6876]
                tunnel: [w6876] -> w6715
                tunnel: w6718 -> [w6885]
                tunnel: w6717 -> [w6884]
                tunnel: w6716 -> [w6882]
                tunnel: w6715 -> [w6883]
                tunnel: w6710 -> [w6881]
                tunnel: w6701 -> [w6880]
                frame #0 {
                  n1984 = while {
                    stop <- w6769 stop-if-true
                    w6770 = 20.0 ("y")
                    n1985 = global read "Robot Global Data.vi" "Distance 2"() -> (w6771:dbl)
                    n1986 = global read "Robot Global Data.vi" "Distance"() -> (w6772:dbl)
                    n1987 = Greater?(x=w6772, y=w6770) -> (0:w6774:bool)
                    n1988 = Greater?(x=w6771, y=w6770) -> (0:w6773:bool)
                    n1989 = And(x=w6774, y=w6773) -> (x .and. y?=w6769:bool)
                    n1990 = global write "Robot Global Data.vi" "Raise_Mast"(w6769) -> ()
                  }
                  n1991 = call "PID Distance.vi"("Distance"=225.0, "Angle"=0.0, "RightEncoder"=w6759, "LeftEncoder"=w6760, "GyroDevRef"=w6761, "RobotDriveDevRef"=w6762) -> ("RightEncoder 2"=w6763:T11, "LeftEncoder 2"=w6764:T11, "GyroDevRef 2"=w6765:T8, "RobotDriveDevRef 2"=w6766:T1)  [unwired: 2 in]
                }
                frame #1 {
                  n1992 = call "PID turning.vi"("Angle"=-90.0, "GyroDevRef"=w6778, "RobotDriveDevRef"=w6777) -> ("GyroDevRef 2"=w6775:T8, "RobotDriveDevRef 2"=w6776:T1)  [unwired: 7 in]
                }
                frame #2 {
                  n1993 = call <vilib>:"WPI_EncoderReset.vi"("EncoderDevRef"=w6787) -> ("EncoderDevRef"=w6785:T11)  [unwired: 9 in, 1 out]
                  n1994 = Wait (ms)(milliseconds to wait=u32 10) -> ()  [unwired: 1 out]
                  n1995 = call <vilib>:"WPI_EncoderReset.vi"("EncoderDevRef"=w6788) -> ("EncoderDevRef"=w6786:T11)  [unwired: 9 in, 1 out]
                }
                frame #3 {
                  n1996 = global read "Robot Global Data.vi" "Axes"() -> (w6800:dbl[])
                  n1997 = call "PID Distance.vi"("Distance"=199.0, "Angle"=-90.0, "RightEncoder"=w6793, "LeftEncoder"=w6794, "GyroDevRef"=w6795, "RobotDriveDevRef"=w6796) -> ("RightEncoder 2"=w6790:T11, "LeftEncoder 2"=w6789:T11, "GyroDevRef 2"=w6792:T8, "RobotDriveDevRef 2"=w6791:T1)  [unwired: 2 in]
                  n1998 = global write "Robot Global Data.vi" "Lift_Position"(2.0) -> ()
                  n1999 = Array To Cluster(array=w6800) -> (cluster=w6799:T15)
                  n2000 = Bundle By Name(cluster=w6799, "Axes[1]"=-1.0) -> (w6798:T15)
                  n2001 = Cluster To Array(cluster=w6798) -> (array=w6797:dbl[])
                  n2002 = global write "Robot Global Data.vi" "Axes"(w6797) -> ()
                }
                frame #4 {
                  n2003 = call "PID turning.vi"("Angle"=0.0, "GyroDevRef"=w6807, "RobotDriveDevRef"=w6808) -> ("GyroDevRef 2"=w6805:T8, "RobotDriveDevRef 2"=w6806:T1)  [unwired: 7 in]
                }
                frame #5 {
                  n2004 = call <vilib>:"WPI_EncoderReset.vi"("EncoderDevRef"=w6813) -> ("EncoderDevRef"=w6816:T11)  [unwired: 9 in, 1 out]
                  n2005 = call <vilib>:"WPI_EncoderReset.vi"("EncoderDevRef"=w6812) -> ("EncoderDevRef"=w6815:T11)  [unwired: 9 in, 1 out]
                }
                frame #6 {
                  n2006 = call "PID Distance.vi"("Distance"=40.0, "Angle"=0.0, "RightEncoder"=w6823, "LeftEncoder"=w6824, "GyroDevRef"=w6826, "RobotDriveDevRef"=w6825) -> ("RightEncoder 2"=w6819:T11, "LeftEncoder 2"=w6820:T11, "GyroDevRef 2"=w6821:T8, "RobotDriveDevRef 2"=w6822:T1)  [unwired: 2 in]
                  n2007 = global write "Robot Global Data.vi" "Lift_Position"(3.0) -> ()
                }
                frame #7 {
                  n2008 = call "PID turning.vi"("Angle"=20.0, "GyroDevRef"=w6830, "RobotDriveDevRef"=w6833) -> ("GyroDevRef 2"=w6829:T8, "RobotDriveDevRef 2"=w6832:T1)  [unwired: 7 in]
                }
                frame #8 {
                  n2009 = call <vilib>:"WPI_EncoderReset.vi"("EncoderDevRef"=w6839) -> ("EncoderDevRef"=w6837:T11)  [unwired: 9 in, 1 out]
                  n2010 = call <vilib>:"WPI_EncoderReset.vi"("EncoderDevRef"=w6838) -> ("EncoderDevRef"=w6836:T11)  [unwired: 9 in, 1 out]
                }
                frame #9 {
                  w6853 = 0.0 ("Left axis value")
                  n2011 = global read "Robot Global Data.vi" "Axes"() -> (w6848:dbl[])
                  n2012 = Wait (ms)(milliseconds to wait=u32 300) -> ()  [unwired: 1 out]
                  n2013 = Array To Cluster(array=w6848) -> (cluster=w6847:T15)
                  n2014 = Bundle By Name(cluster=w6847, "Axes[1]"=0.25) -> (w6850:T15)
                  n2015 = Cluster To Array(cluster=w6850) -> (array=w6849:dbl[])
                  n2016 = call <vilib>:"WPI_RobotDriveTankDrive.vi"("Right axis value"=w6853, "Left axis value"=w6853, "RobotDriveDevRef"=w6852) -> ("RobotDriveDevRef"=w6846:T1)  [unwired: 6 in, 2 out]
                  n2017 = global write "Robot Global Data.vi" "Axes"(w6849) -> ()
                }
                frame #10 {
                  n2018 = global write "Robot Global Data.vi" "Current State"(FALSE ("Current State")) -> ()
                  n2019 = Wait (ms)(milliseconds to wait=u32 400) -> ()  [unwired: 1 out]
                }
                frame #11 {
                  n2020 = global read "Robot Global Data.vi" "Axes"() -> (w6870:dbl[])
                  n2021 = call "PID Distance.vi"("Distance"=-20.0, "Angle"=20.0, "RightEncoder"=w6871, "LeftEncoder"=w6872, "GyroDevRef"=w6860, "RobotDriveDevRef"=w6861) -> ("RightEncoder 2"=w6862:T11, "LeftEncoder 2"=w6863:T11, "GyroDevRef 2"=w6864:T8, "RobotDriveDevRef 2"=w6865:T1)  [unwired: 2 in]
                  n2022 = Array To Cluster(array=w6870) -> (cluster=w6869:T15)
                  n2023 = Bundle By Name(cluster=w6869, "Axes[1]"=-1.0) -> (w6868:T15)
                  n2024 = Cluster To Array(cluster=w6868) -> (array=w6867:dbl[])
                  n2025 = global write "Robot Global Data.vi" "Axes"(w6867) -> ()
                }
                frame #12 {
                  n2026 = global write "Robot Global Data.vi" "Lift_Position"(1.0) -> ()
                }
                frame #13 {
                  n2027 = case shown="\"R\"" w6881 {
                    tunnel: w6885 -> [w6898 w6977 _]
                    tunnel: w6884 -> [w6897 w6976 _]
                    tunnel: w6883 -> [w6896 w6974 _]
                    tunnel: w6882 -> [w6895 w6975 _]
                    tunnel: w6880 -> [w6886 w6961 _]
                    frame "R" {
                      n2028 = flat-sequence {
                        tunnel: w6898 -> [w6907]
                        tunnel: w6897 -> [w6906]
                        tunnel: [w6909] -> w6904
                        tunnel: [w6908] -> w6903
                        tunnel: w6904 -> [w6916]
                        tunnel: w6903 -> [w6915]
                        tunnel: [w6916] -> w6899
                        tunnel: [w6915] -> w6900
                        tunnel: [w6913] -> w6901
                        tunnel: [w6912] -> w6902
                        tunnel: w6896 -> [w6911]
                        tunnel: w6895 -> [w6910]
                        tunnel: w6902 -> [w6917]
                        tunnel: w6901 -> [w6918]
                        tunnel: w6900 -> [w6921]
                        tunnel: w6899 -> [w6922]
                        tunnel: [w6920] -> w6894
                        tunnel: [w6919] -> w6892
                        tunnel: [w6918] -> w6890
                        tunnel: [w6917] -> w6888
                        tunnel: w6894 -> [w6950]
                        tunnel: [w6950] -> w6893
                        tunnel: w6892 -> [w6949]
                        tunnel: [w6949] -> w6891
                        tunnel: w6890 -> [w6948]
                        tunnel: [w6946] -> w6889
                        tunnel: w6888 -> [w6947]
                        tunnel: [w6945] -> w6887
                        tunnel: w6893 -> [w6955]
                        tunnel: w6891 -> [w6954]
                        tunnel: w6889 -> [w6953]
                        tunnel: w6887 -> [w6952]
                        tunnel: w6886 -> [w6951]
                        frame #0 {
                          n2029 = call "PID turning.vi"("Angle"=170.0, "GyroDevRef"=w6906, "RobotDriveDevRef"=w6907) -> ("GyroDevRef 2"=w6908:T8, "RobotDriveDevRef 2"=w6909:T1)  [unwired: 7 in]
                        }
                        frame #1 {
                          n2030 = call <vilib>:"WPI_EncoderReset.vi"("EncoderDevRef"=w6910) -> ("EncoderDevRef"=w6913:T11)  [unwired: 9 in, 1 out]
                          n2031 = Wait (ms)(milliseconds to wait=u32 10) -> ()  [unwired: 1 out]
                          n2032 = call <vilib>:"WPI_EncoderReset.vi"("EncoderDevRef"=w6911) -> ("EncoderDevRef"=w6912:T11)  [unwired: 9 in, 1 out]
                        }
                        frame #2 {
                          n2033 = global read "Robot Global Data.vi" "Axes"() -> (w6929:dbl[])
                          n2034 = Wait (ms)(milliseconds to wait=u32 400) -> ()  [unwired: 1 out]
                          n2035 = Array To Cluster(array=w6929) -> (cluster=w6930:T15)
                          n2036 = global read "Robot Global Data.vi" "PIXY Output"() -> (w6923:T16)
                          n2037 = Bundle By Name(cluster=w6930, "Axes[1]"=1.0) -> (w6931:T15)
                          n2038 = Unbundle By Name(w6923) -> ("SIGNATURE NUMBER"=w6926:u16)
                          n2039 = global read "Robot Global Data.vi" "Cube Signature"() -> (w6925:dbl)
                          n2040 = Equal?(x=w6926, y=w6925) -> (x = y?=w6924:bool)
                          n2041 = Cluster To Array(cluster=w6931) -> (array=w6932:dbl[])
                          n2042 = global write "Robot Global Data.vi" "Axes"(w6932) -> ()
                          n2043 = case shown="False" w6924 {
                            tunnel: [w6939 w6942] -> w6919
                            tunnel: [w6940 w6941] -> w6920
                            tunnel: w6922 -> [w6934 w6941]
                            tunnel: w6921 -> [w6933 w6942]
                            frame True {
                              n2044 = call <vilib>:"WPI_GyroGetAngle.vi"("GyroDevRef"=w6933) -> ("Angle"=w6938:dbl, "GyroDevRef"=w6939:T8)  [unwired: 6 in, 3 out]
                              n2045 = In Range and Coerce(upper limit=170.0, x=w6938, lower limit=110.0) -> (coerced(x)=w6937:dbl)  [unwired: 1 out]
                              n2046 = global write "Robot Global Data.vi" "Tracked Angle"(w6937) -> ()
                              n2047 = call "PID vision.vi"("RobotDriveDevRef in"=w6934) -> ("RobotDriveDevRef out"=w6940:T1)  [unwired: 9 in, 1 out]
                            }
                            frame False {
                              n2048 = global write "Robot Global Data.vi" "Tracked Angle"(170.0) -> ()
                            }
                          }
                        }
                        frame #3 {
                          n2049 = call <vilib>:"WPI_EncoderReset.vi"("EncoderDevRef"=w6948) -> ("EncoderDevRef"=w6946:T11)  [unwired: 9 in, 1 out]
                          n2050 = Wait (ms)(milliseconds to wait=u32 10) -> ()  [unwired: 1 out]
                          n2051 = call <vilib>:"WPI_EncoderReset.vi"("EncoderDevRef"=w6947) -> ("EncoderDevRef"=w6945:T11)  [unwired: 9 in, 1 out]
                        }
                        frame #4 {
                          n2052 = global read "Robot Global Data.vi" "Tracked Angle"() -> (w6956:dbl)
                          n2053 = call "PID with Infrared.vi"("RobotDriveDevRef"=w6955, "Angle"=w6956, "Encoder Limit"=60.0 ("Distance"), "GyroDevRef"=w6954, "Left Encoder"=w6952, "Right Encoder"=w6953, "DigitalInputDevRef"=w6951) -> ()  [unwired: 4 in, 5 out]
                        }
